vi "TangoGroup.vi"() -> ()   [LabVIEW 2013, in "examples.lvlib"]
uses:
  examples.lvlib
  vis/lv-2013/tango_vi.llb/avToShortScalar.vi
  vis/lv-2013/tango_vi.llb/avToDoubleScalar.vi
  vis/lv-2013/tango_vi.llb/tango.lvlib
panel:
  out "values":T1(array[cluster])
  out "Waveform Chart":dbl(graph)=2.864694317803e-312
  out "Waveform Chart":i16(graph)=74
  in  "?":bool
  out "attribute name":string
  out "attribute name":string
  out "device name":string
  out "device name":string
  in  "attribute names (will be read on each group member)":string[](array[string])=["short_scalar", "double_scalar"]
  out "group id":i32=42
  in  "group name":string="test_group"
  in  "managed devices":string[](array[string])=["sys/tg_test/1", "sys/tg_test/2"]
  in  "ignored devices":string[](array[string])
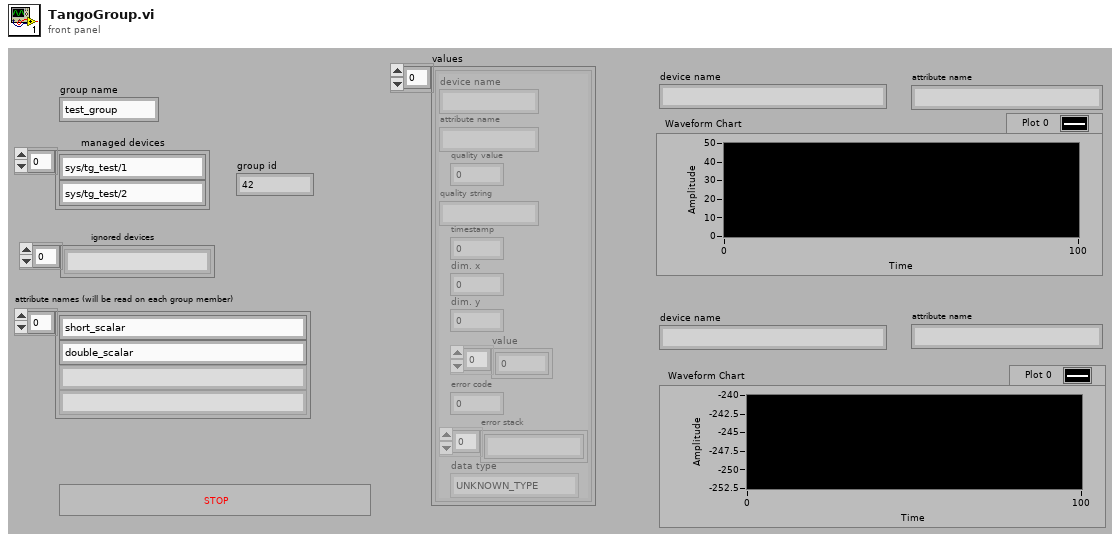
[diagram p1: front panel]
types:
  T1 = cluster{"device name":string, "attribute name":string, "quality value":i16, "quality string":string, "timestamp":dbl, "dim. x":i32, "dim. y":i32, "value":u8[], "error code":i32, "error stack":string[], "data type":enum16{"SCA_STATE", "SCA_STRING", "SPE_STRING", "IMG_STRING", "SCA_BOOLEAN", "SPE_BOOLEAN", "IMG_BOOLEAN", "SCA_UCHAR", "SPE_UCHAR", "IMG_UCHAR", "SCA_SHORT", "SPE_SHORT", "IMG_SHORT", "SCA_USHORT", "SPE_USHORT", "IMG_USHORT", "SCA_LONG", "SPE_LONG", "IMG_LONG", "SCA_ULONG", "SPE_ULONG", "IMG_ULONG", "SCA_FLOAT", "SPE_FLOAT", "IMG_FLOAT", "SCA_DOUBLE", "SPE_DOUBLE", "IMG_DOUBLE", "UNKNOWN_TYPE"}}[]
  T2 = cluster{"device name":string, "attribute name":string, "quality value":i16, "quality string":string, "timestamp":dbl, "dim. x":i32, "dim. y":i32, "value":u8[], "error code":i32, "error stack":string[], "data type":u16}[]
  T3 = cluster{"device name":string, "attribute name":string, "quality value":i16, "quality string":string, "timestamp":dbl, "dim. x":i32, "dim. y":i32, "value":u8[], "error code":i32, "error stack":string[], "data type":u16}
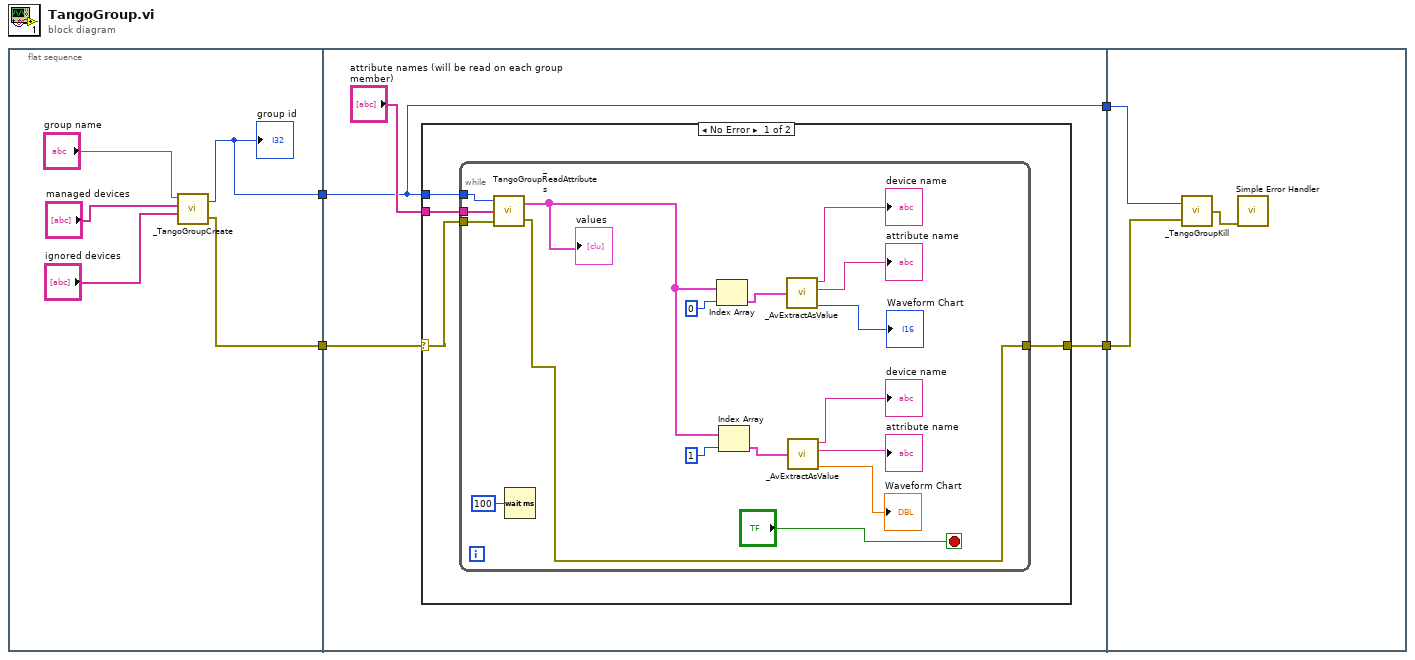
[diagram p0: block diagram]
diagram:
  n1 = flat-sequence {
    tunnel: [w8] -> w4
    tunnel: [w7] -> w2
    tunnel: w4 -> [w12]
    tunnel: [w12] -> w3
    tunnel: w2 -> [w11]
    tunnel: [w10] -> w1
    tunnel: w3 -> [w38]
    tunnel: w1 -> [w37]
    frame #0 {
      n2 = call "_TangoGroupCreate.vi"("ignored devices"="ignored devices", "managed devices"="managed devices", "group name"="group name") -> ("error out"=w7:errorcluster, "group id"=w8:i32)  [unwired: 1 in]
      "group id" <- w8
    }
    frame #1 {
      n3 = case shown="No Error" w11 {
        selector: w11 -> [w15 w35]
        tunnel: "attribute names (will be read on each group member)" -> [w17 _]
        tunnel: w12 -> [w16 _]
        tunnel: [w14 w35] -> w10
        frame No Error {
          n4 = while {
            tunnel: w17 -> [w34]
            tunnel: w16 -> [w33]
            tunnel: w15 -> [w19]
            tunnel: [w18] -> w14
            stop <- "?" stop-if-true
            n5 = call "_TangoGroupReadAttributes.vi"("error in"=w19, "attribute names"=w34, "group id"=w33) -> ("error out"=w18:errorcluster, "values"=w25:T2)
            "values" <- w25
            n6 = Wait (ms)(milliseconds to wait=u32 100) -> ()  [unwired: 1 out]
            n7 = Index Array(array=w25, index=0 ("indice")) -> (element=w20:T3)
            n8 = Index Array(array=w25, index=1 ("indice")) -> (element=w21:T3)
            n9 = call-poly "_AvExtractAsValue.vi"("attribute value"=w20) -> ("value"=→"Waveform Chart":i16, "attribute name"=→"attribute name":string, "device name"=→"device name":string)  [unwired: 2 out]
            n10 = call-poly "_AvExtractAsValue.vi"("attribute value"=w21) -> ("value"=→"Waveform Chart":dbl, "attribute name"=→"attribute name":string, "device name"=→"device name":string)  [unwired: 2 out]
          }
        }
        frame Error {
        }
      }
    }
    frame #2 {
      n11 = call "_TangoGroupKill.vi"("error in"=w37, "group id"=w38) -> ("error out"=w36:errorcluster)
      n12 = call <vilib>:"Simple Error Handler.vi"("error in (no error)"=w36) -> ()  [unwired: 4 in, 5 out]
    }
  }
